vi "Set Initialization Data - gRPC Server.vi"(8 "error in":errorcluster, 11 "Head_ScopeSim in":refnum<class "Head_ScopeSim.lvclass">) -> (0 "error out":errorcluster, 3 "Head_ScopeSim out":refnum<class "Head_ScopeSim.lvclass">)   [LabVIEW 2019, in "Head_ScopeSim.lvclass"]
doc: "In this VI you can set the initialization data of a statically-linked subWorker."
uses:
  Head_ScopeSim.lvclass
  gRPC Server/gRPC Server/gRPC Server.lvclass
  <vilib>/addons/_Workers/Library/Case Label.ctl
  <vilib>/addons/_Workers/Library/Workers.lvlib
  gRPC Server/gRPC Server/Response Cases.ctl
  gRPC Server/gRPC Server/Initialization Data.ctl
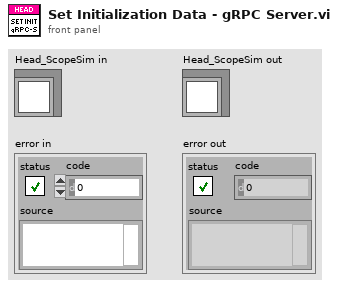
[diagram p1: front panel]
types:
  T1 = typedef "gRPC Server (scope.proto).lvlib/gRPC Server.lvclass/Initialization Data.ctl" = cluster{"Response Cases":T2}
  T2 = typedef "gRPC Server (scope.proto).lvlib/gRPC Server.lvclass/Response Cases.ctl" = cluster{"Connection Notify":T3, "Server Error":T3, "Msg_ToServer_1":T3, "Msg_ToServer_2":T3, "Msg_ToServer_3":T3, "Msg_ToServer_4":T3, "Msg_ToServer_5":T3, "Msg_ToServer_6":T3, "Msg_ToServer_7":T3, "Msg_ToServer_8":T3, "Msg_ToServer_9":T3}
  T3 = typedef "Workers.lvlib/Case Label.ctl" = string
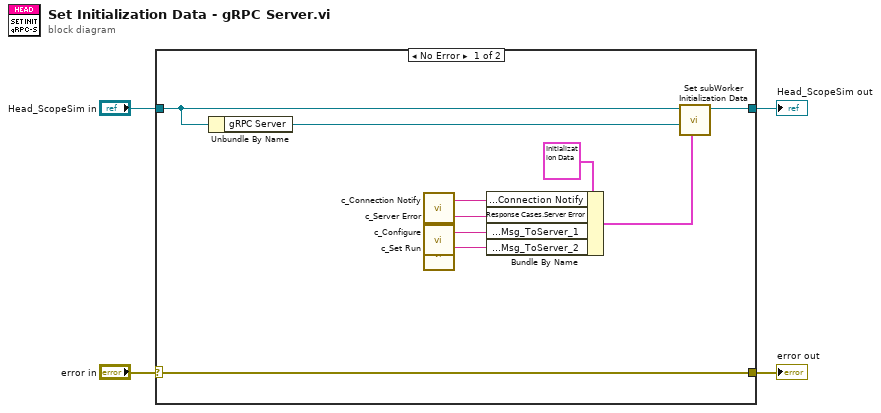
[diagram p0: block diagram]
diagram:
  n1 = case shown="No Error" "error in" {
    selector: "error in" -> [w14 w16]
    tunnel: [w14 w16] -> w3
    tunnel: [w12 w15] -> w2
    tunnel: "Head_ScopeSim in" -> [w11 w15]
    frame No Error {
      n2 = Unbundle By Name(w11) -> ("gRPC Server"=w13:refnum<class "gRPC Server.lvclass">)
      n3 = call "c_Connection Notify.vi"() -> ("Case Label"=w7:T3)  [unwired: 1 in]
      n4 = call "c_Server Error.vi"() -> ("Case Label"=w6:T3)  [unwired: 1 in]
      n5 = call "c_Configure.vi"() -> ("Case Label"=w5:T3)  [unwired: 1 in]
      n6 = call "c_Set Run.vi"() -> ("Case Label"=w8:T3)  [unwired: 1 in]
      n7 = Bundle By Name(cluster=T1 {"Response Cases"={"Connection Notify"="", "Server Error"="", "Msg_ToServer_1"="", "Msg_ToServer_2"="", "Msg_ToServer_3"="", "Msg_ToServer_4"="", "Msg_ToServer_5"="", "Msg_ToServer_6"="", "Msg_ToServer_7"="", "Msg_ToServer_8"="", "Msg_ToServer_9"=""}} ("Initialization Data"), "Response Cases.Connection Notify"=w7, "Response Cases.Server Error"=w6, "Response Cases.Msg_ToServer_1"=w5, "Response Cases.Msg_ToServer_2"=w8) -> (w9:T1)
      n8 = call-dynamic "Set subWorker Initialization Data.vi"("Initialization Data"=w9, "subWorker"=w13, "Worker"=w11) -> ("Worker out"=w12:refnum<class "Head_ScopeSim.lvclass">)  [unwired: 8 in]
    }
    frame Error {
    }
  }
  "error out" <- w3
  "Head_ScopeSim out" <- w2
